vi "Wait for home.vi"(8 "error in (no error)":errorcluster, 11 "VISA Refnum in":refnum<visa-resource-name>) -> (0 "error out":errorcluster, 3 "VISA resource name out":refnum<visa-resource-name>)   [LabVIEW 2020]
uses:
  Public/Controls/Motor direction.ctl
  Public/Controls/Move motor parameters--cluster.ctl
  Public/Controls/Step style.ctl
  Public/Write--move.vi
  Public/Write--home.vi
  Control de MaP.lvlib
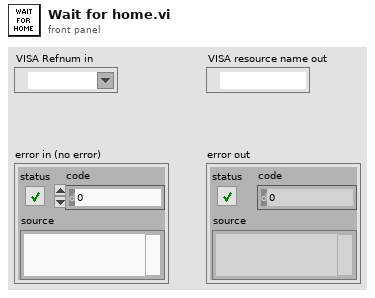
[diagram p1: front panel]
types:
  T1 = typedef "Control de MaP.lvlib/Move motor parameters--cluster.ctl" = cluster{"Action":u8, "Direction motor 1":T2, "Direction motor 2":T2, "Steps motor 1":u16, "Steps motor 2":u16, "Step style motor 1":T3, "Step style motor 2":T3}
  T2 = typedef "Control de MaP.lvlib/Motor direction.ctl" = u8
  T3 = typedef "Control de MaP.lvlib/Step style.ctl" = u8
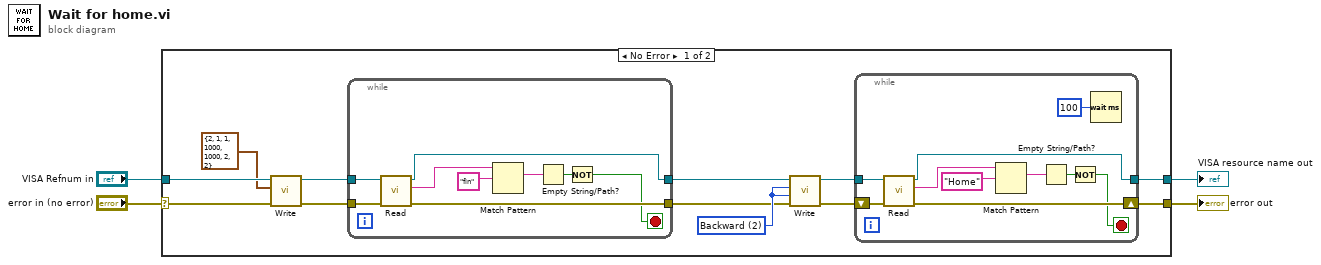
[diagram p0: block diagram]
diagram:
  n1 = case shown="No Error" "error in (no error)" {
    selector: "error in (no error)" -> [w11 w37]
    tunnel: [w16 w37] -> w4
    tunnel: [w15 w36] -> w3
    tunnel: "VISA Refnum in" -> [w10 w36]
    frame No Error {
      w12 = T2 2 items=["", "Forward", "Backward"] ("Home direction")
      n2 = call-poly "Write.vi"("error in (no error)"=w11, "Comando"=T1 {"Action"=2, "Direction motor 1"=1, "Direction motor 2"=1, "Steps motor 1"=1000, "Steps motor 2"=1000, "Step style motor 1"=2, "Step style motor 2"=2}, "VISA resource name"=w10) -> ("error out"=w7:errorcluster, "VISA resource name out"=w9:refnum<visa-resource-name>)  [unwired: 6 in, 1 out]
      n3 = while {
        tunnel: w9 -> [w21]
        tunnel: [w17] -> w8
        tunnel: w7 -> [w20]
        tunnel: [w19] -> w6
        stop <- w18 stop-if-true
        n4 = call "Read.vi"("error in (no error)"=w20, "VISA resource name"=w21) -> ("error out"=w19:errorcluster, "Recibo de Datos"=w22:string, "VISA resource name out"=w17:refnum<visa-resource-name>)  [unwired: 6 in, 1 out]
        n5 = Match Pattern(string=w22, regular expression="fin") -> (match substring=w24:string)  [unwired: 1 in, 3 out]
        n6 = Empty String/Path?(string/path=w24) -> (empty?=w23:bool)
        n7 = Not(x=w23) -> (.not. x?=w18:bool)
      }
      n8 = call-poly "Write.vi"("error in (no error)"=w6, "Home direction (M2)"=w12, "Home direction (M1)"=w12, "VISA resource name"=w8) -> ("error out"=w14:errorcluster, "VISA resource name out"=w13:refnum<visa-resource-name>)  [unwired: 4 in, 2 out]
      n9 = while {
        shift-right: [w34] -> w16
        shift-left: w14 -> [w35]
        tunnel: w13 -> [w33]
        tunnel: [w27] -> w15
        stop <- w28 stop-if-true
        n10 = call "Read.vi"("error in (no error)"=w35, "VISA resource name"=w33) -> ("error out"=w34:errorcluster, "Recibo de Datos"=w29:string, "VISA resource name out"=w27:refnum<visa-resource-name>)  [unwired: 6 in, 1 out]
        n11 = Match Pattern(string=w29, regular expression="Home") -> (match substring=w31:string)  [unwired: 1 in, 3 out]
        n12 = Empty String/Path?(string/path=w31) -> (empty?=w30:bool)
        n13 = Not(x=w30) -> (.not. x?=w28:bool)
        n14 = Wait (ms)(milliseconds to wait=u32 100) -> ()  [unwired: 1 out]
      }
    }
    frame Error {
    }
  }
  "error out" <- w4
  "VISA resource name out" <- w3
